vi "MultirunBuilder.vi"() -> ()   [LabVIEW 2022 SP3]
uses:
  Anemometry Sub Vis/File/Setup_Filetype.ctl
  Anemometry Sub Vis/Globals/Meas_global.vi
  Anemometry Sub Vis/Controls/Multi_run_mode.ctl
  Anemometry Sub Vis/Gen Trav/Spacing.ctl
  MultirunBuilderSubVIs/Single Measurement.vi
  MultirunBuilderSubVIs/Set Speed Only.vi
  MultirunBuilderSubVIs/Auto Calibrate.vi
  MultirunBuilderSubVIs/MoveTTcall.vi
  Anemometry Sub Vis/Controls/Tunnel_Coordinates.ctl
  MultirunBuilderSubVIs/Wait (minutes).vi
  <vilib>/Platform/system.llb/System Exec.vi
  <vilib>/Platform/browser.llb/Open URL in Default Browser (path).vi
  MultirunBuilderSubVIs/RowTemplate.ctl
  MultirunBuilderSubVIs/ReformattedTaskArray.ctl
panel:
  in  "Open Cmd File":bool
  in  "Generate Cmd File":bool
  in  "Tab Control":enum32{"Globals", "Task Array", "Dev"}(tab)
  in  "TaskArray":T1 {"Carrier_2 Q (l/min)" format="%#.2f"; "Row Duration (mins)" format="%#.1f min"; "Row No" min=0 format="row %.0f"; "Trace Gas Concentration (%)" min=0.0 format="%#_4f"; "Carrier_1 Q (l/min)" format="%#.2f"; "Tunnel Speed" format="%#.2f m/s"; "Start X" format="%#.2f"; "Start Y" format="%#.2f"; "Start Z" format="%#.2f"; "End X" format="%#.2f"; "End Y" format="%#.2f"; "End Z" format="%#.2f"; "No. of pts." format="%.0f pts"; "Averaging time (min)" min=0.0 format="%#.2f min"}
  out "Startup Index":bool
  in  "Re-initialize":bool
  in  "Stop Button":bool
  in  "RowTemplate":T3 {"Carrier_2 Q (l/min)" format="%#.2f"; "Row Duration (mins)" format="%#.1f"; "Row No" min=0; "Trace Gas Concentration (%)" min=0.0 format="%#_4f"; "Carrier_1 Q (l/min)" format="%#.2f"; "Tunnel Speed" format="%#.2f"; "Start X" format="%#.2f"; "Start Y" format="%#.2f"; "Start Z" format="%#.2f"; "End X" format="%#.2f"; "End Y" format="%#.2f"; "End Z" format="%#.2f"; "Averaging time (min)" min=0.0 format="%#.2f"}
  # "X           Y            Z"
  # "Start"
  # "End"
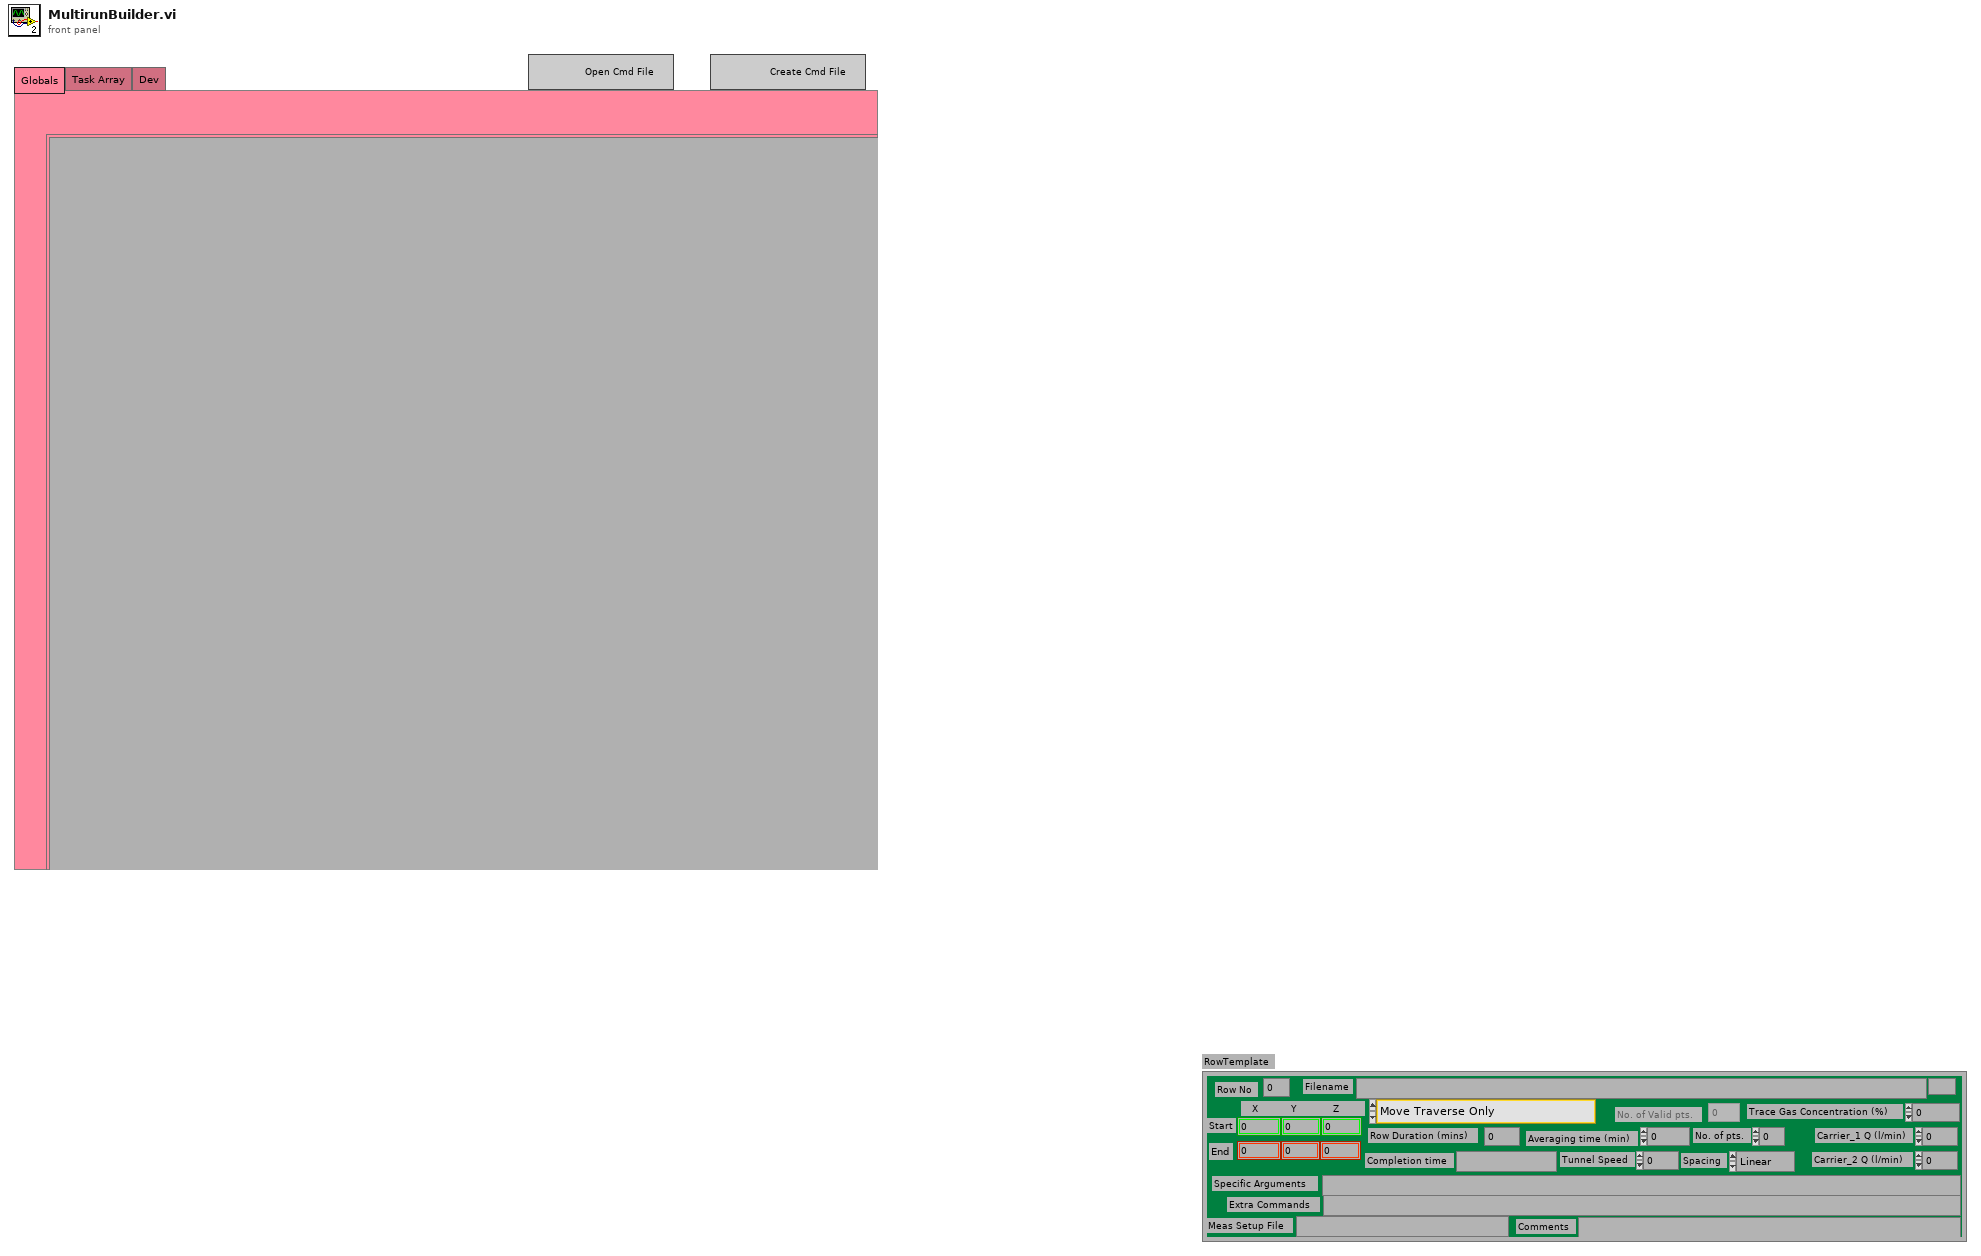
[diagram p1: front panel]
types:
  T1 = typedef "ReformattedTaskArray.ctl" = cluster{"Start X":sgl, "Start Y":sgl, "Start Z":sgl, "End X":sgl, "End Y":sgl, "End Z":sgl, "No. of pts.":i32, "Spacing":T2, "Filename":path, "Tunnel Speed":dbl, "Averaging time (min)":dbl, "Extra Commands":string, "Carrier_1 Q (l/min)":dbl, "Carrier_2 Q (l/min)":dbl, "Trace Gas Concentration (%)":dbl, "Specific Arguments":string, "Comments":string, "Row No":i32, "Row Type Selector":enum16{"Move Traverse Only", "Set Tunnel Speed Only", "Set Source Only", "Set Measurement Conditions", "Single Measurement", "Vertical Profile", "Lateral Profile", "Longitudinal Profile", "Explore Volume", "Multi-Axis Profile", "Auto Calibrate", "Meas Fast FID Bkgnd", "Check Beam Power", "Scanning Valve Measurement", "Run VI Named:", "Set ADAM Ch", "Wait (minutes)", "Send Message", "Synchronize With:", "Fall Back to this Row", "Turn Off Row Repeating", "Blank Row", "Traverse 3D Volume"}, "Completion time":string, "Row Duration (mins)":dbl, "No. of Valid pts.":i32, "Meas Setup File":string}[]
  T2 = typedef "Spacing.ctl" = enum16{"Linear", "Log", "Gauss", "Specified", "N/A"}
  T3 = typedef "RowTemplate.ctl" = cluster{"Start X":sgl, "Start Y":sgl, "Start Z":sgl, "End X":sgl, "End Y":sgl, "End Z":sgl, "No. of pts.":i32, "Spacing":T2, "Filename":path, "Tunnel Speed":dbl, "Averaging time (min)":dbl, "Extra Commands":string, "Carrier_1 Q (l/min)":dbl, "Carrier_2 Q (l/min)":dbl, "Trace Gas Concentration (%)":dbl, "Specific Arguments":string, "Comments":string, "Row No":i32, "Row Type Selector":T4, "Completion time":string, "Row Duration (mins)":dbl, "No. of Valid pts.":i32, "Meas Setup File":string}
  T4 = typedef "Multi_run_mode.ctl" = enum16{"Move Traverse Only", "Set Tunnel Speed Only", "Set Source Only", "Set Measurement Conditions", "Single Measurement", "Vertical Profile", "Lateral Profile", "Longitudinal Profile", "Multi-Axis Profile", "Explore Volume", "Auto Calibrate", "Meas Fast FID Bkgnd", "Check Beam Power", "Scanning Valve Measurement", "Run VI Named:", "Set ADAM Ch", "Wait (minutes)", "Send Message", "Synchronize With:", "Fall Back to this Row", "Turn Off Row Repeating", "Traverse 3D Volume", "Blank Row", "Jump to Fall Back Row"}
  T5 = cluster{"Azimuth Array Index":u32, "Vert Prof Array Index":u32, "Lat Prof Array Index":u32, "Azimuth Array Index 2":u32}
  T6 = enum16{"Load Command File", "Save Command File", "Check Multi Run Prog", "Check Multi Run Prog With Live Moves", "Run Multi Run Prog"}
  T7 = typedef "Tunnel_Coordinates.ctl" = enum16{"Work in Tunnel Coordinates", "Work in Model Coordinates"}
  T8 = cluster{"Tunnel Warm Up":bool, "AutoCal":bool, "Zeroes 2":bool, "Turn Table Schedule":bool, "Global Cal Checks":bool, "Local Cal Checks":bool, "Vertical Profile":bool, "Lateral Profile":bool, "Reinitialize Task Array":bool, "Save Command File":bool, "Longitudinal Profile":bool}
  T9 = typedef "CorrectionsCluster.ctl" = cluster{"Use Height Corrections":bool, "TT.Azimuths":dbl[], "Z.HeightCorrs":dbl[][], "Corrections from File":bool, "Height Survey Filepaths":path[]}
  T10 = cluster{"Start X":sgl, "Start Y":sgl, "Start Z":sgl, "End X":sgl, "End Y":sgl, "End Z":sgl, "No. of pts.":i32, "Spacing":T2, "Filename":path, "Tunnel Speed":dbl, "Averaging time (min)":dbl, "Extra Commands":string, "Carrier_1 Q (l/min)":dbl, "Carrier_2 Q (l/min)":dbl, "Trace Gas Concentration (%)":dbl, "Specific Arguments":string, "Comments":string, "Row No":i32, "Row Type Selector":T4, "Completion time":string, "Row Duration (mins)":dbl, "No. of Valid pts.":i32, "Meas Setup File":string}[]
  T11 = cluster{"Start X":sgl, "Start Y":sgl, "Start Z":sgl, "End X":sgl, "End Y":sgl, "End Z":sgl, "No. of pts.":i32, "Spacing":T2, "Filename":path, "Tunnel Speed":dbl, "Averaging time (min)":dbl, "Extra Commands":string, "Carrier_1 Q (l/min)":dbl, "Carrier_2 Q (l/min)":dbl, "Trace Gas Concentration (%)":dbl, "Specific Arguments":string, "Comments":string, "Row No":i32, "Row Type Selector":u16, "Completion time":string, "Row Duration (mins)":dbl, "No. of Valid pts.":i32, "Meas Setup File":string}[]
  T12 = typedef "SingleMeas_Repeater.ctl" = cluster{"X":dbl, "Y":dbl, "Z":dbl, "Use Tunnel Coords?":bool, "RepeatEveryXDeg":dbl}
  T13 = cluster{"Tunnel Speed":dbl, "X":dbl, "Y":dbl, "Z":dbl, "Comments":string, "Use Tunnel Coords?":bool}
  T14 = cluster{"Velocity (m/s)":dbl, "X":dbl, "Y":dbl, "Z":dbl, "Comments":string, "Use Tunnel Coords?":bool}
  T15 = typedef "MRBRowTaskSelector.ctl" = enum16{"Move Traverse Only", "Set Tunnel Speed Only", "Set Source Only", "Set Measurement Conditions", "Single Measurement", "Vertical Profile", "Lateral Profile", "Longitudinal Profile", "Explore Volume", "Multi-Axis Profile", "Auto Calibrate", "Meas Fast FID Bkgnd", "Check Beam Power", "Scanning Valve Measurement", "Run VI Named:", "MoveTT", "TravZSurvey", "Set ADAM Ch", "Wait (minutes)", "Send Message", "Synchronize With:", "Fall Back to this Row", "Turn Off Row Repeating", "Blank Row", "Traverse 3D Volume"}
  T16 = cluster{"Row Type Selector":T15, "Index":dbl, "Direction":enum16{"Forward", "Reverse"}}[]
  T17 = cluster{"Tunnel Off":bool, "Local Cal Checks":bool, "Global Cal Checks":bool, "Zeroes":bool, "AutoCal":bool, "Turn Table --> Zero":bool}
  T18 = typedef "Setup_Filetype.ctl" = enum16{"Measurement Setups", "Calibration Setups", "General", "Results File Plotter Setups", "Speed Calib Tweaks"}
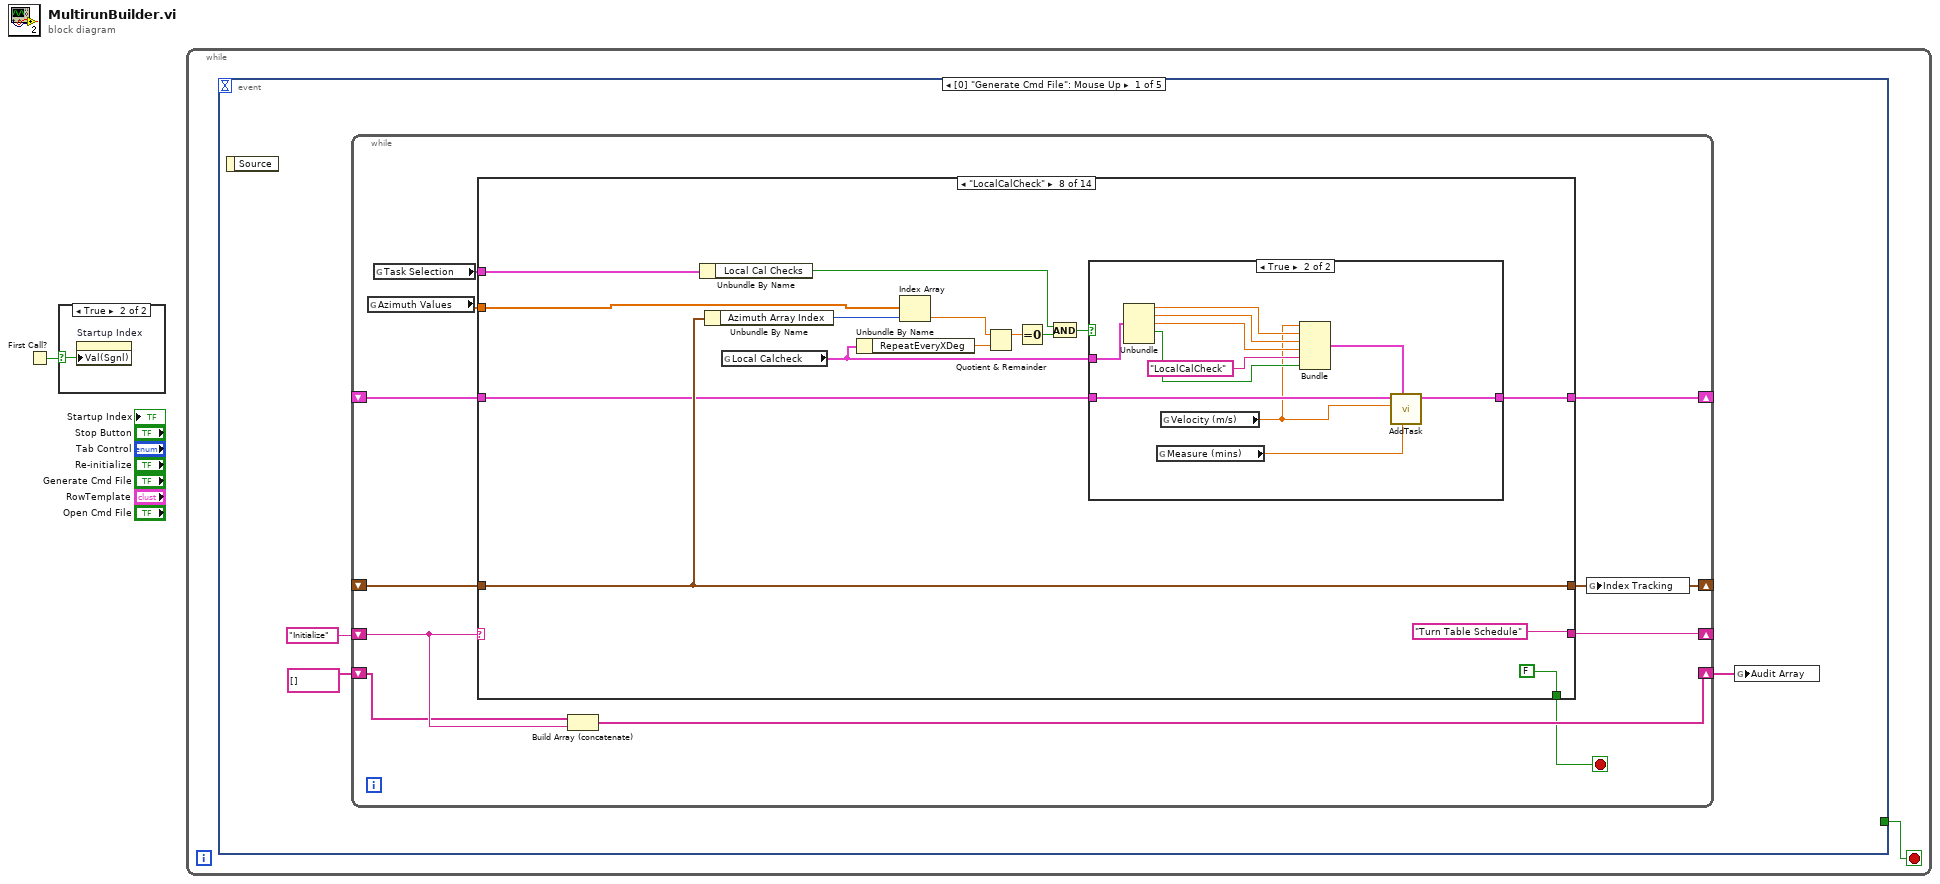
[diagram p0: block diagram]
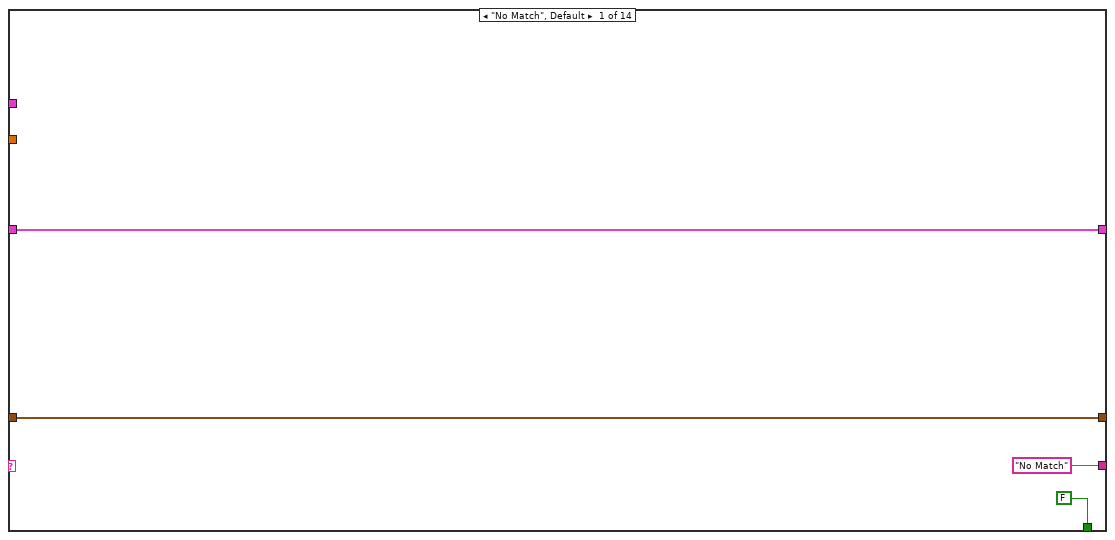
[diagram p2: hidden frame]
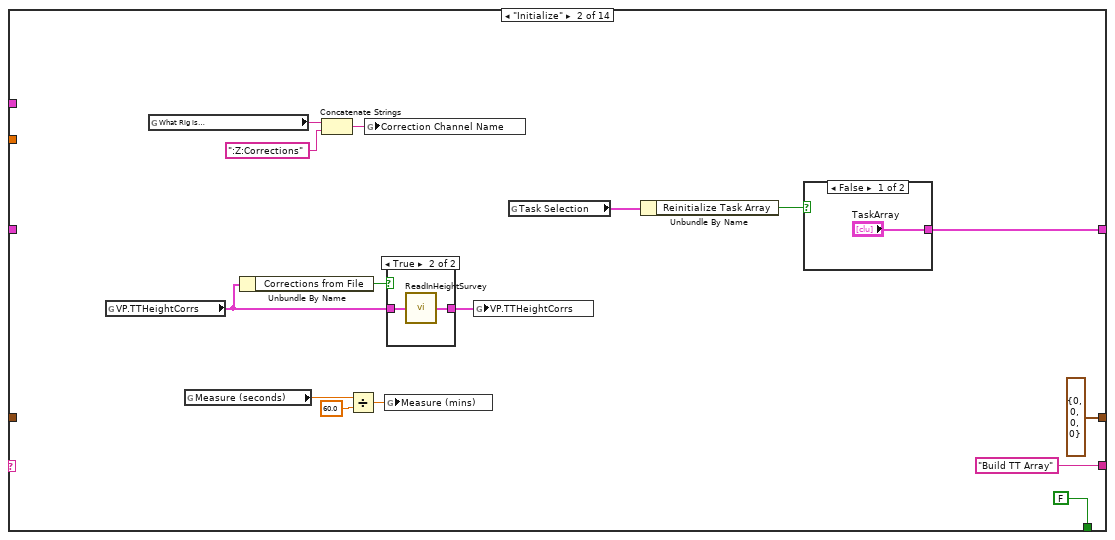
[diagram p3: hidden frame]
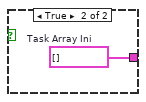
[diagram p5: hidden frame]
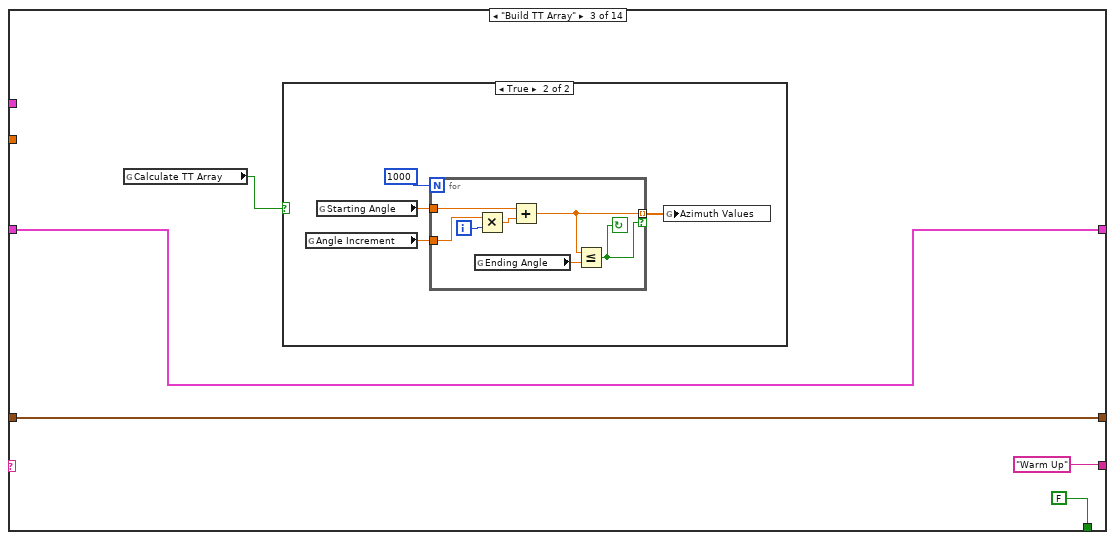
[diagram p6: hidden frame]
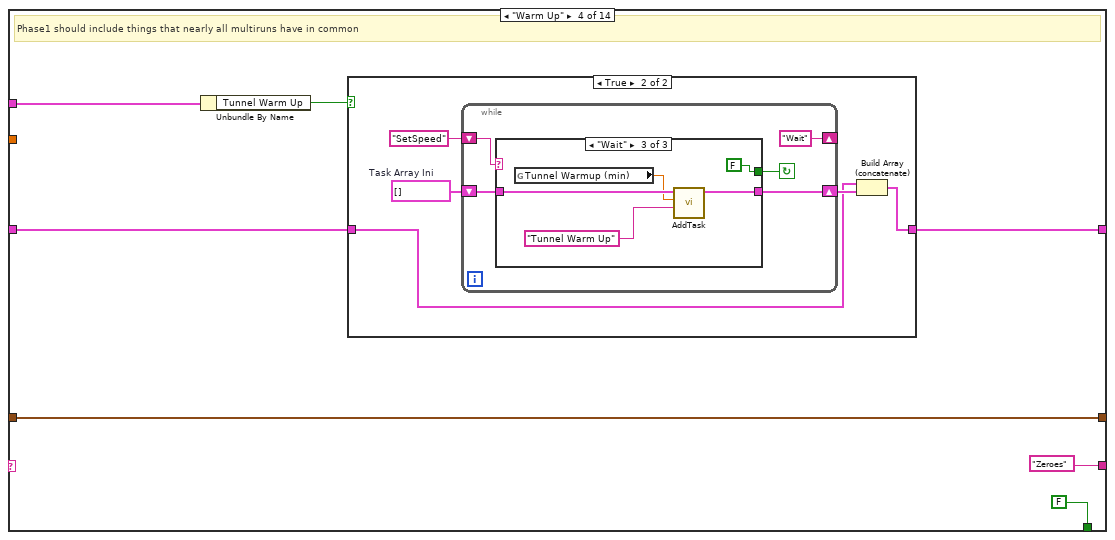
[diagram p8: hidden frame]
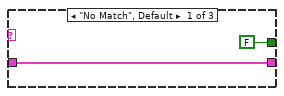
[diagram p10: hidden frame]
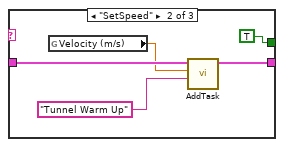
[diagram p11: hidden frame]
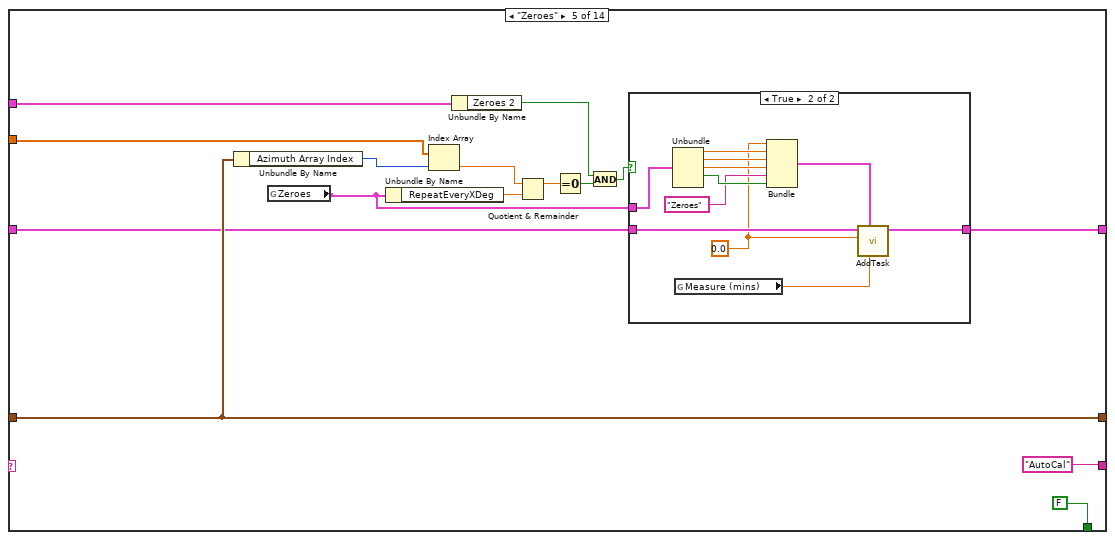
[diagram p12: hidden frame]
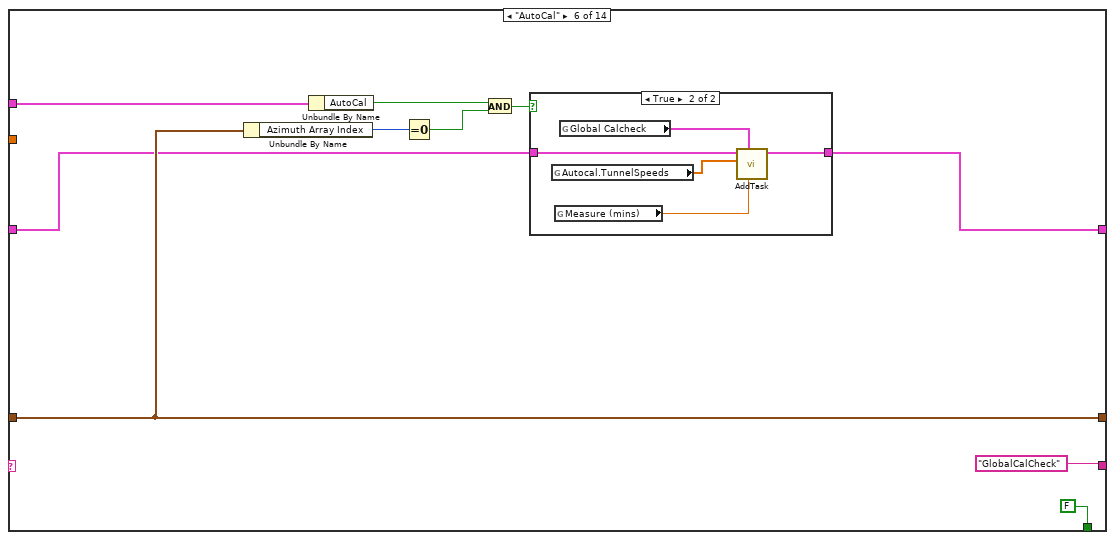
[diagram p14: hidden frame]
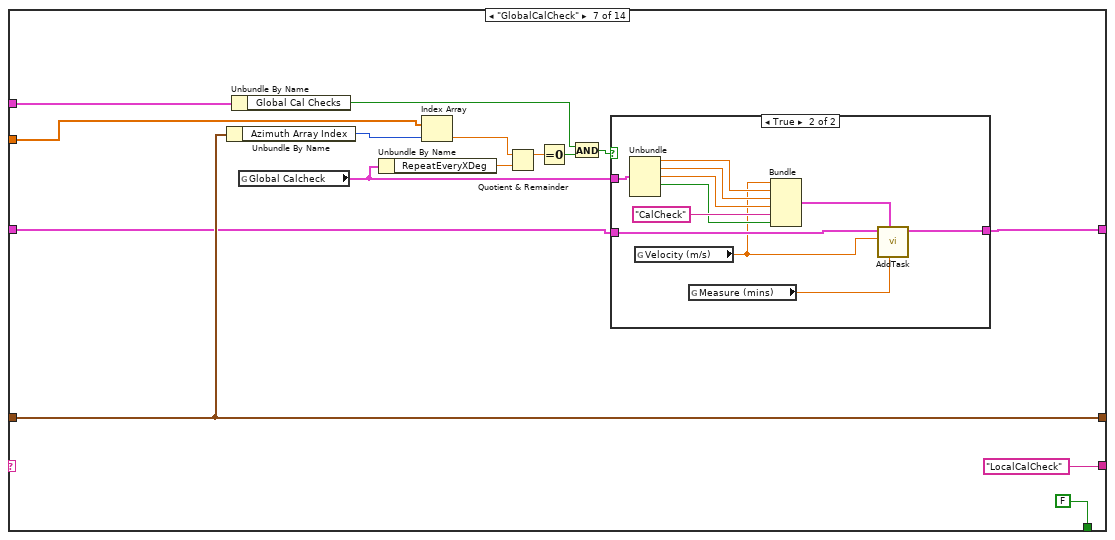
[diagram p16: hidden frame]
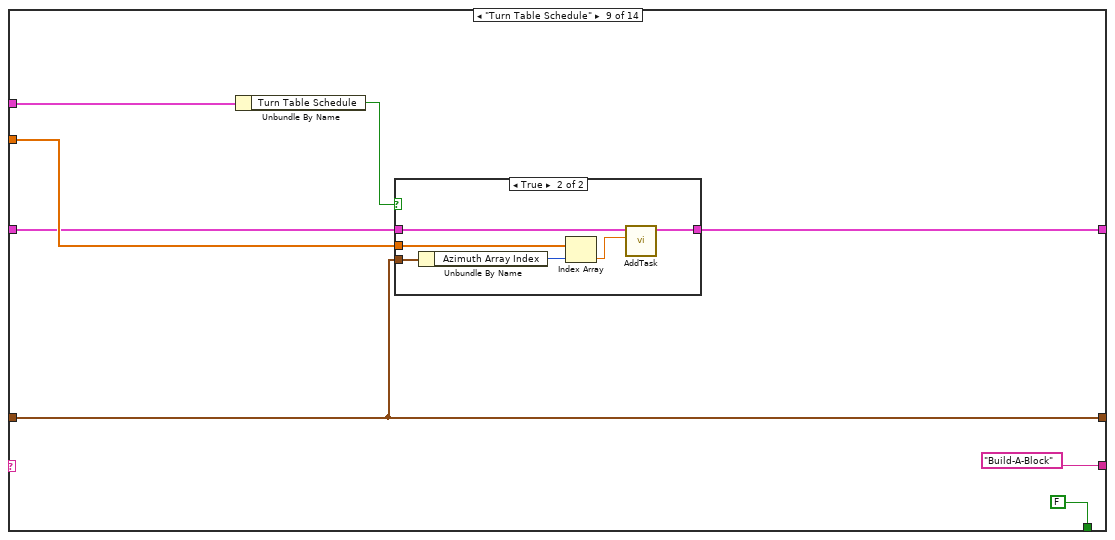
[diagram p19: hidden frame]
diagram:
  n1 = First Call?() -> (First Call?: T/F=w1:bool)
  n2 = case shown="True" w1 {
    selector: w1 -> [_ w2]
    frame False {
    }
    frame True {
      n3 = property on="Startup Index" class="Bool (strict)"("Val(Sgnl)"=w2) -> ()  [unwired: 2 in, 2 out]
    }
  }
  n4 = while {
    stop <- w3 stop-if-true
    n5 = event shown="[0] \"Generate Cmd File\": Mouse Up" {
      selector: _ -> [_ _ _ _ _]
      dyn-events: _ -> [_ _ _ _ _]
      timeout: _ -> [_ _ _ _ _]
      tunnel: [_ _ _ _ TRUE] -> w3
      event "Generate Cmd File": Mouse Up {
        n6 = event-data() -> ()  [unwired: 1 in, 1 out]
        n7 = while {
          shift-right: [w17] -> _
          shift-left: "Initialize" -> [w15]
          shift-right: [w10] -> _
          shift-left: _ -> [w11]
          shift-right: [w14] -> w6
          shift-left: string[] [] -> [w13]
          shift-right: [w9] -> _
          shift-left: _ -> [w16]
          stop <- w12 stop-if-true
          n8 = global read "MRCMDFBGlobal.vi" "Azimuth Values"() -> (w7:dbl[])
          n9 = global read "MRCMDFBGlobal.vi" "Task Selection"() -> (w8:T8)
          n10 = case shown="\"LocalCalCheck\"" w15 {
            tunnel: ["No Match" "Build TT Array" "Warm Up" "Zeroes" "AutoCal" "GlobalCalCheck" "LocalCalCheck" "Turn Table Schedule" "Build-A-Block" "Repeat?" w211 "Save Multirun?" ("t") "Last Chance for Stuff" ("t") _] -> w17
            tunnel: [FALSE ("Stop Button") FALSE ("Stop Button") FALSE ("Stop Button") FALSE ("Stop Button") FALSE ("Stop Button") FALSE ("Stop Button") FALSE ("Stop Button") FALSE ("Stop Button") FALSE ("Stop Button") FALSE ("Stop Button") FALSE ("Stop Button") FALSE FALSE TRUE ("Stop Button")] -> w12
            tunnel: w7 -> [_ _ _ _ w100 _ w135 w161 w191 _ w210 _ _ _]
            tunnel: w16 -> [w19 _ w45 w62 w98 w121 w138 w166 w187 w201 w216 w244 w342 w364]
            tunnel: [w19 T5 {"Azimuth Array Index"=0, "Vert Prof Array Index"=0, "Lat Prof Array Index"=0, "Azimuth Array Index 2"=0} ("Index Tracking") w45 w62 w98 w121 w138 w166 w187 w201 w214 w244 w342 w364] -> w9
            tunnel: w8 -> [_ _ _ w61 w94 w117 w137 w165 w188 _ w207 _ w346 _]
            tunnel: w11 -> [w18 _ w43 w59 w89 w115 w132 w160 w186 w203 w208 w235 w344 w363]
            tunnel: [w18 w31 w43 w58 w90 w116 w133 w159 w185 w202 w208 w236 w340 w363] -> w10
            frame "No Match", Default {
            }
            frame "Initialize" {
              n11 = global read "MRCMDFBGlobal.vi" "VP.TTHeightCorrs"() -> (w28:T9)
              n12 = global read "MRCMDFBGlobal.vi" "What Rig is\nMultirunning?"() -> (w24:string)
              n13 = global read "MRCMDFBGlobal.vi" "Measure (seconds)"() -> (w25:dbl)
              n14 = Unbundle By Name(w28) -> ("Corrections from File"=w30:bool)
              n15 = Concatenate Strings(w24, ":Z:Corrections") -> (w22:string)
              n16 = Divide(x=w25, y=60.0 ("x")) -> (x/y=w26:dbl)
              n17 = global write "MRCMDFBGlobal.vi" "Correction Channel Name"(w22) -> ()
              n18 = global write "MRCMDFBGlobal.vi" "Measure (mins)"(w26) -> ()
              n19 = case shown="True" w30 {
                tunnel: w28 -> [w37 w39]
                tunnel: [w37 w38] -> w29
                frame False {
                }
                frame True {
                  n20 = call "ReadInHeightSurvey.vi"("VP.TTHeightCorrs In"=w39) -> ("VP.TTHeightCorrs Out"=w38:T9)
                }
              }
              n21 = global write "MRCMDFBGlobal.vi" "VP.TTHeightCorrs"(w29) -> ()
              n22 = global read "MRCMDFBGlobal.vi" "Task Selection"() -> (w33:T8)
              n23 = Unbundle By Name(w33) -> ("Reinitialize Task Array"=w32:bool)
              n24 = case shown="False" w32 {
                tunnel: ["TaskArray" w41] -> w31
                frame False {
                }
                frame True {
                  w41 = T10 []  # Task Array Ini
                }
              }
            }
            frame "Build TT Array" {
              n25 = global read "MRCMDFBGlobal.vi" "Calculate TT Array"() -> (w42:bool)
              n26 = case shown="True" w42 {
                frame False {
                }
                frame True {
                  n27 = global read "MRCMDFBGlobal.vi" "Angle Increment"() -> (w47:dbl)
                  n28 = global read "MRCMDFBGlobal.vi" "Starting Angle"() -> (w48:dbl)
                  n29 = for {
                    N: 1000 -> [_]
                    tunnel: w48 -> [w55]
                    tunnel: w47 -> [w56]
                    tunnel: [w53] -> w49 mode=indexing if=w52
                    i -> [w57]
                    stop <- w52 continue-if-true
                    n30 = global read "MRCMDFBGlobal.vi" "Ending Angle"() -> (w51:dbl)
                    n31 = Multiply(x=w56, y=w57) -> (x*y=w54:dbl)
                    n32 = Add(x=w55, y=w54) -> (x+y=w53:dbl)
                    n33 = Less Or Equal?(x=w53, y=w51) -> (x <= y?=w52:bool)
                  }
                  n34 = global write "MRCMDFBGlobal.vi" "Azimuth Values"(w49) -> ()
                }
              }
            }
            frame "Warm Up" {
              # "Phase1 should include things that nearly all multiruns have in common"
              n35 = Unbundle By Name(w61) -> ("Tunnel Warm Up"=w60:bool)
              n36 = case shown="True" w60 {
                tunnel: w59 -> [w65 w67]
                tunnel: [w65 w66] -> w58
                frame False {
                }
                frame True {
                  w69 = T10 []  # Task Array Ini
                  n37 = while {
                    shift-right: ["Wait"] -> _
                    shift-left: "SetSpeed" -> [w75]
                    shift-right: [w71] -> w68
                    shift-left: w69 -> [w72]
                    stop <- w73 continue-if-true
                    n38 = case shown="\"Wait\"" w75 {
                      tunnel: [FALSE TRUE FALSE] -> w73
                      tunnel: w72 -> [w76 w80 w85]
                      tunnel: [w76 w79 w84] -> w71
                      frame "No Match", Default {
                      }
                      frame "SetSpeed" {
                        n39 = global read "MRCMDFBGlobal.vi" "Velocity (m/s)"() -> (w78:dbl)
                        n40 = call-poly "AddTask.vi"("Comments"="Tunnel Warm Up", "Tunnel Speed"=w78, "Input Task Array"=w80) -> ("Output Task Array"=w79:T3[])  [unwired: 8 in]
                      }
                      frame "Wait" {
                        n41 = global read "MRCMDFBGlobal.vi" "Tunnel Warmup (min)"() -> (w83:dbl)
                        n42 = call-poly "AddTask.vi"("Comments"="Tunnel Warm Up", "Wait Time (min)"=w83, "Input Task Array"=w85) -> ("Output Task Array"=w84:T3[])  [unwired: 8 in]
                      }
                    }
                  }
                  n43 = Build Array (concatenate)(w67, w68) -> (w66:T11)
                }
              }
            }
            frame "Zeroes" {
              n44 = Unbundle By Name(w98) -> ("Azimuth Array Index"=w99:u32)
              n45 = global read "MRCMDFBGlobal.vi" "Zeroes"() -> (w88:T12)
              n46 = Unbundle By Name(w88) -> ("RepeatEveryXDeg"=w96:dbl)
              n47 = Index Array(array=w100, index=w99) -> (element=w97:dbl)
              n48 = Unbundle By Name(w94) -> ("Zeroes 2"=w93:bool)
              n49 = Quotient & Remainder(x=w97, y=w96) -> (x-y*floor(x/y)=w95:dbl)  [unwired: 1 out]
              n50 = Equal To 0?(x=w95) -> (x = 0?=w92:bool)
              n51 = And(x=w93, y=w92) -> (x .and. y?=w91:bool)
              n52 = case shown="True" w91 {
                tunnel: w88 -> [_ w112]
                tunnel: [w103 w114] -> w90
                tunnel: w89 -> [w103 w113]
                frame False {
                }
                frame True {
                  w104 = 0.0 ("Tunnel Speed")
                  n53 = Unbundle(w112) -> ("X"=w111:dbl, "Y"=w110:dbl, "Z"=w109:dbl, "Use Tunnel Coords?"=w107:bool)  [unwired: 1 out]
                  n54 = global read "MRCMDFBGlobal.vi" "Measure (mins)"() -> (w105:dbl)
                  n55 = Bundle("Tunnel Speed"=w104, "X"=w111, "Y"=w110, "Z"=w109, "Comments"="Zeroes", "Use Tunnel Coords?"=w107) -> (w108:T13)  [unwired: 1 in]
                  n56 = call-poly "AddTask.vi"("Averaging time (min)"=w105, "Coordinate Description"=w108, "Tunnel Speed"=w104, "Input Task Array"=w113) -> ("Output Task Array"=w114:T3[])  [unwired: 7 in]
                }
              }
            }
            frame "AutoCal" {
              n57 = Unbundle By Name(w121) -> ("Azimuth Array Index"=w120:u32)
              n58 = Unbundle By Name(w117) -> ("AutoCal"=w119:bool)
              n59 = Equal To 0?(x=w120) -> (x = 0?=w122:bool)
              n60 = And(x=w119, y=w122) -> (x .and. y?=w118:bool)
              n61 = case shown="True" w118 {
                tunnel: [w125 w130] -> w116
                tunnel: w115 -> [w125 w129]
                frame False {
                }
                frame True {
                  n62 = global read "MRCMDFBGlobal.vi" "Autocal.TunnelSpeeds"() -> (w128:dbl[])
                  n63 = global read "MRCMDFBGlobal.vi" "Measure (mins)"() -> (w127:dbl)
                  n64 = global read "MRCMDFBGlobal.vi" "Global Calcheck"() -> (w126:T12)
                  n65 = call-poly "AddTask.vi"("Averaging time (min)"=w127, "Global Calcheck"=w126, "Autocal.TunnelSpeeds"=w128, "Input Task Array"=w129) -> ("Output Task Array"=w130:T3[])  [unwired: 7 in]
                }
              }
            }
            frame "GlobalCalCheck" {
              n66 = Unbundle By Name(w138) -> ("Azimuth Array Index"=w143:u32)
              n67 = Unbundle By Name(w137) -> ("Global Cal Checks"=w136:bool)
              n68 = global read "MRCMDFBGlobal.vi" "Global Calcheck"() -> (w131:T12)
              n69 = Unbundle By Name(w131) -> ("RepeatEveryXDeg"=w141:dbl)
              n70 = Index Array(array=w135, index=w143) -> (element=w142:dbl)
              n71 = Quotient & Remainder(x=w142, y=w141) -> (x-y*floor(x/y)=w140:dbl)  [unwired: 1 out]
              n72 = Equal To 0?(x=w140) -> (x = 0?=w139:bool)
              n73 = And(x=w136, y=w139) -> (x .and. y?=w134:bool)
              n74 = case shown="True" w134 {
                tunnel: w131 -> [_ w155]
                tunnel: [w146 w157] -> w133
                tunnel: w132 -> [w146 w156]
                frame False {
                }
                frame True {
                  n75 = Unbundle(w155) -> ("X"=w153:dbl, "Y"=w152:dbl, "Z"=w151:dbl, "Use Tunnel Coords?"=w150:bool)  [unwired: 1 out]
                  n76 = global read "MRCMDFBGlobal.vi" "Velocity (m/s)"() -> (w147:dbl)
                  n77 = global read "MRCMDFBGlobal.vi" "Measure (mins)"() -> (w148:dbl)
                  n78 = Bundle("Velocity (m/s)"=w147, "X"=w153, "Y"=w152, "Z"=w151, "Comments"="CalCheck", "Use Tunnel Coords?"=w150) -> (w149:T14)  [unwired: 1 in]
                  n79 = call-poly "AddTask.vi"("Averaging time (min)"=w148, "Coordinate Description"=w149, "Tunnel Speed"=w147, "Input Task Array"=w156) -> ("Output Task Array"=w157:T3[])  [unwired: 7 in]
                }
              }
            }
            frame "LocalCalCheck" {
              n80 = Unbundle By Name(w165) -> ("Local Cal Checks"=w164:bool)
              n81 = Unbundle By Name(w166) -> ("Azimuth Array Index"=w170:u32)
              n82 = global read "MRCMDFBGlobal.vi" "Local Calcheck"() -> (w158:T12)
              n83 = Unbundle By Name(w158) -> ("RepeatEveryXDeg"=w168:dbl)
              n84 = Index Array(array=w161, index=w170) -> (element=w169:dbl)
              n85 = Quotient & Remainder(x=w169, y=w168) -> (x-y*floor(x/y)=w167:dbl)  [unwired: 1 out]
              n86 = Equal To 0?(x=w167) -> (x = 0?=w163:bool)
              n87 = And(x=w164, y=w163) -> (x .and. y?=w162:bool)
              n88 = case shown="True" w162 {
                tunnel: w158 -> [_ w182]
                tunnel: w160 -> [w173 w184]
                tunnel: [w173 w183] -> w159
                frame False {
                }
                frame True {
                  n89 = Unbundle(w182) -> ("X"=w176:dbl, "Y"=w177:dbl, "Z"=w178:dbl, "Use Tunnel Coords?"=w179:bool)  [unwired: 1 out]
                  n90 = global read "MRCMDFBGlobal.vi" "Measure (mins)"() -> (w175:dbl)
                  n91 = global read "MRCMDFBGlobal.vi" "Velocity (m/s)"() -> (w174:dbl)
                  n92 = Bundle("Velocity (m/s)"=w174, "X"=w176, "Y"=w177, "Z"=w178, "Comments"="LocalCalCheck", "Use Tunnel Coords?"=w179) -> (w180:T14)  [unwired: 1 in]
                  n93 = call-poly "AddTask.vi"("Averaging time (min)"=w175, "Coordinate Description"=w180, "Tunnel Speed"=w174, "Input Task Array"=w184) -> ("Output Task Array"=w183:T3[])  [unwired: 7 in]
                }
              }
            }
            frame "Turn Table Schedule" {
              n94 = Unbundle By Name(w188) -> ("Turn Table Schedule"=w189:bool)
              n95 = case shown="True" w189 {
                tunnel: w191 -> [_ w199]
                tunnel: w187 -> [_ w198]
                tunnel: w186 -> [w193 w197]
                tunnel: [w193 w196] -> w185
                frame False {
                }
                frame True {
                  n96 = Unbundle By Name(w198) -> ("Azimuth Array Index"=w195:u32)
                  n97 = Index Array(array=w199, index=w195) -> (element=w194:dbl)
                  n98 = call-poly "AddTask.vi"("TT:Azimuth"=w194, "Input Task Array"=w197) -> ("Output Task Array"=w196:T3[])  [unwired: 9 in]
                }
              }
            }
            frame "Build-A-Block" {
              n99 = global read "MRCMDFBGlobal.vi" "Build-A-Block"() -> (w200:T16)
              n100 = call "MR_Build-A-Block.vi"("Build-A-Block"=w200) -> ("TaskArray"=w204:T10)
              n101 = Build Array (concatenate)(w203, w204) -> (w202:T11)
            }
            frame "Repeat?" {
              # "Only reason to repeat is if TT Scheduling"
              n102 = Unbundle By Name(w207) -> ("Turn Table Schedule"=w209:bool)
              n103 = case shown="True" w209 {
                tunnel: w216 -> [w218 w225]
                tunnel: [TRUE w224] -> w215
                tunnel: [w218 w223] -> w214
                tunnel: w210 -> [_ w222]
                frame False {
                }
                frame True {
                  n104 = Array Size(array=w222) -> (size(s)=w221:i32)
                  n105 = Decrement(x=w221) -> (x-1=w220:i32)
                  n106 = in-place {
                    in-place-border: w220 -> [w227]
                    in-place-border: [w228] -> w224
                    n107 = in-place-cluster #1(w225) -> ("Azimuth Array Index"=w226:u32)
                    n108 = Equal?(x=w227, y=w226) -> (x = y?=w228:bool)
                    n109 = case shown="True" w228 {
                      tunnel: [w230 0] -> w229
                      tunnel: w226 -> [w231 _]
                      frame False {
                        n110 = Increment(x=w231) -> (x+1=w230:u32)
                      }
                      frame True {
                      }
                    }
                    n111 = in-place-cluster #1("Azimuth Array Index"=w229) -> (w223:T5)
                  }
                }
              }
              n112 = Select(t="End", s=w215, f="Zeroes" ("t")) -> (s? t:f=w211:string)
            }
            frame "End" {
              n113 = global read "MRCMDFBGlobal.vi" "Multirun Closure Tasks"() -> (w233:T17)
              n114 = Unbundle By Name(w233) -> ("Turn Table --> Zero"=w242:bool, "Zeroes"=w241:bool, "AutoCal"=w240:bool, "Global Cal Checks"=w239:bool, "Local Cal Checks"=w238:bool, "Tunnel Off"=w237:bool)
              n115 = while {
                shift-right: [w255] -> _
                shift-left: "Turn Table" -> [w256]
                tunnel: w242 -> [w254]
                tunnel: w241 -> [w251]
                tunnel: w240 -> [w250]
                tunnel: w239 -> [w249]
                tunnel: w238 -> [w248]
                tunnel: w237 -> [w247]
                shift-right: [w252] -> w236
                shift-left: w235 -> [w253]
                stop <- w246 continue-if-true
                n116 = case shown="\"Zeroes\"" w256 {
                  tunnel: [_ "Zeroes" "AutoCal" "GlobalCalCheck" "LocalCalCheck" "Tunnel Off" _] -> w255
                  tunnel: w254 -> [_ w263 _ _ _ _ _]
                  tunnel: w253 -> [w258 w262 w272 w289 w300 w317 w333]
                  tunnel: [w258 w261 w271 w288 w299 w316 w332] -> w252
                  tunnel: w251 -> [_ _ w268 _ _ _ _]
                  tunnel: w250 -> [_ _ _ w285 _ _ _]
                  tunnel: w249 -> [_ _ _ _ w297 _ _]
                  tunnel: w248 -> [_ _ _ _ _ w314 _]
                  tunnel: w247 -> [_ _ _ _ _ _ w331]
                  tunnel: [FALSE TRUE TRUE TRUE TRUE TRUE TRUE] -> w246
                  frame "No Match", Default {
                  }
                  frame "Turn Table" {
                    n117 = case shown="True" w263 {
                      tunnel: w262 -> [w264 w266]
                      tunnel: [w264 w265] -> w261
                      frame False {
                      }
                      frame True {
                        n118 = call-poly "AddTask.vi"("TT:Azimuth"=0.0, "Input Task Array"=w266) -> ("Output Task Array"=w265:T3[])  [unwired: 9 in]
                      }
                    }
                  }
                  frame "Zeroes" {
                    n119 = case shown="True" w268 {
                      tunnel: w272 -> [w273 w284]
                      tunnel: [w273 w283] -> w271
                      frame False {
                      }
                      frame True {
                        w274 = 0.0 ("Tunnel Speed")
                        n120 = global read "MRCMDFBGlobal.vi" "Zeroes"() -> (w275:T12)
                        n121 = global read "MRCMDFBGlobal.vi" "Measure (mins)"() -> (w276:dbl)
                        n122 = Unbundle(w275) -> ("X"=w281:dbl, "Y"=w280:dbl, "Z"=w279:dbl, "Use Tunnel Coords?"=w278:bool)  [unwired: 1 out]
                        n123 = Bundle("Tunnel Speed"=w274, "X"=w281, "Y"=w280, "Z"=w279, "Comments"="Zeroes", "Use Tunnel Coords?"=w278) -> (w277:T13)  [unwired: 1 in]
                        n124 = call-poly "AddTask.vi"("Averaging time (min)"=w276, "Coordinate Description"=w277, "Tunnel Speed"=w274, "Input Task Array"=w284) -> ("Output Task Array"=w283:T3[])  [unwired: 7 in]
                      }
                    }
                  }
                  frame "AutoCal" {
                    n125 = case shown="True" w285 {
                      tunnel: w289 -> [w290 w295]
                      tunnel: [w290 w294] -> w288
                      frame False {
                      }
                      frame True {
                        n126 = global read "MRCMDFBGlobal.vi" "Autocal.TunnelSpeeds"() -> (w293:dbl[])
                        n127 = global read "MRCMDFBGlobal.vi" "Global Calcheck"() -> (w291:T12)
                        n128 = global read "MRCMDFBGlobal.vi" "Measure (mins)"() -> (w292:dbl)
                        n129 = call-poly "AddTask.vi"("Averaging time (min)"=w292, "Global Calcheck"=w291, "Autocal.TunnelSpeeds"=w293, "Input Task Array"=w295) -> ("Output Task Array"=w294:T3[])  [unwired: 7 in]
                      }
                    }
                  }
                  frame "GlobalCalCheck" {
                    n130 = case shown="True" w297 {
                      tunnel: w300 -> [w301 w312]
                      tunnel: [w301 w311] -> w299
                      frame False {
                      }
                      frame True {
                        n131 = global read "MRCMDFBGlobal.vi" "Global Calcheck"() -> (w304:T12)
                        n132 = global read "MRCMDFBGlobal.vi" "Measure (mins)"() -> (w303:dbl)
                        n133 = global read "MRCMDFBGlobal.vi" "Velocity (m/s)"() -> (w302:dbl)
                        n134 = Unbundle(w304) -> ("X"=w308:dbl, "Y"=w307:dbl, "Z"=w306:dbl, "Use Tunnel Coords?"=w305:bool)  [unwired: 1 out]
                        n135 = Bundle("Velocity (m/s)"=w302, "X"=w308, "Y"=w307, "Z"=w306, "Comments"="CalCheck", "Use Tunnel Coords?"=w305) -> (w309:T14)  [unwired: 1 in]
                        n136 = call-poly "AddTask.vi"("Averaging time (min)"=w303, "Coordinate Description"=w309, "Tunnel Speed"=w302, "Input Task Array"=w312) -> ("Output Task Array"=w311:T3[])  [unwired: 7 in]
                      }
                    }
                  }
                  frame "LocalCalCheck" {
                    n137 = case shown="True" w314 {
                      tunnel: w317 -> [w318 w329]
                      tunnel: [w318 w328] -> w316
                      frame False {
                      }
                      frame True {
                        n138 = global read "MRCMDFBGlobal.vi" "Local Calcheck"() -> (w321:T12)
                        n139 = global read "MRCMDFBGlobal.vi" "Velocity (m/s)"() -> (w319:dbl)
                        n140 = global read "MRCMDFBGlobal.vi" "Measure (mins)"() -> (w320:dbl)
                        n141 = Unbundle(w321) -> ("X"=w327:dbl, "Y"=w326:dbl, "Z"=w325:dbl, "Use Tunnel Coords?"=w322:bool)  [unwired: 1 out]
                        n142 = Bundle("Velocity (m/s)"=w319, "X"=w327, "Y"=w326, "Z"=w325, "Comments"="LocalCalCheck", "Use Tunnel Coords?"=w322) -> (w323:T14)  [unwired: 1 in]
                        n143 = call-poly "AddTask.vi"("Averaging time (min)"=w320, "Coordinate Description"=w323, "Tunnel Speed"=w319, "Input Task Array"=w329) -> ("Output Task Array"=w328:T3[])  [unwired: 7 in]
                      }
                    }
                  }
                  frame "Tunnel Off" {
                    n144 = case shown="True" w331 {
                      tunnel: w333 -> [w334 w336]
                      tunnel: [w334 w335] -> w332
                      frame False {
                      }
                      frame True {
                        n145 = call-poly "AddTask.vi"("Comments"="Tunnel Off", "Tunnel Speed"=0.0, "Input Task Array"=w336) -> ("Output Task Array"=w335:T3[])  [unwired: 8 in]
                      }
                    }
                  }
                }
              }
            }
            frame "Save Multirun?" {
              n146 = Unbundle By Name(w346) -> ("Save Command File"=w345:bool)
              n147 = global read "MRCMDFBGlobal.vi" "Command File Path / Name"() -> (w341:path)
              n148 = case shown="True" w345 {
                tunnel: w341 -> [_ w352]
                tunnel: w344 -> [w347 w349]
                tunnel: [w347 w349] -> w340
                frame False {
                }
                frame True {
                  n149 = global read "MRCMDFBGlobal.vi" "Work in TUNNEL Coordinates"() -> (w348:bool)
                  n150 = case shown="False" w348 {
                    tunnel: [Tunnel_Coordinates."Work in Model Coordinates" ("Work in Tunnel Coordinates?") Tunnel_Coordinates."Work in Tunnel Coordinates" ("Work in Tunnel Coordinates?")] -> w350
                    frame False {
                    }
                    frame True {
                    }
                  }
                  n151 = call "Multi_Run_Prog.vi"("Command filename"=w352, "Mode"=T6."Save Command File", "Table"=w349, "Work in Tunnel Coordinates?"=w350) -> ()  [unwired: 15 in, 1 out]
                }
              }
              n152 = local write "TaskArray"(w340) -> ()
            }
            frame "Last Chance for Stuff" {
              n153 = vi-ref "Multi_Run_Prog.vi"() -> (w356:refnum<vi>)
              n154 = property class="VI"(reference=w356) -> (error out=w359:errorcluster, "Panel"=w357:refnum<vi>)  [unwired: 1 in, 1 out]
              n155 = property class="Pnl"(reference=w357, error in=w359) -> (error out=w360:errorcluster, "Controls[]"=w358:refnum<vi>[])  [unwired: 1 out]
              n156 = for {
                tunnel: w358 -> [w370] mode=indexing
                tunnel: [w369] -> w361 if=w368
                tunnel: w360 -> [w367]
                stop <- w368 stop-if-true
                n157 = property class="Ctl"(reference=w370, error in=w367) -> (reference out=w371:refnum<vi>, error out=w366:errorcluster, "Label.Text"=w372:string)
                n158 = property class="Ctl"(reference=w371, error in=w366) -> ("Value"=w369:variant)  [unwired: 2 out]
                n159 = Equal?(x=w372, y="Command filename") -> (x = y?=w368:bool)
              }
              n160 = Variant To Data(type=path "", Variant=w361) -> (data=w355:path)  [unwired: 1 in, 1 out]
              n161 = global write "MRCMDFBGlobal.vi" "Command File Path / Name"(w355) -> ()
            }
          }
          n162 = Build Array (concatenate)(w13, w15) -> (w14:string[])
          n163 = global write "MRCMDFBGlobal.vi" "Index Tracking"(w9) -> ()
        }
        n164 = global write "MRCMDFBGlobal.vi" "Audit Array"(w6) -> ()
      }
      event "Re-initialize": Mouse Up; "Startup Index": Value Change {
        n165 = event-data() -> ()  [unwired: 1 in, 4 out]
        n166 = while {
          shift-right: [w376] -> _
          shift-left: "Load Subpanel" -> [w377]
          stop <- w375 stop-if-true
          n167 = case shown="\"Meas Setups\"" w377 {
            tunnel: ["End" "End" "End" "Meas Setups"] -> w376
            tunnel: [TRUE _ TRUE _] -> w375
            frame "No Match", Default {
            }
            frame "Meas Setups" {
              n168 = disable-structure shown="Enabled" {
                frame Disabled {
                  w383 = Setup_Filetype."Measurement Setups" ("Setup File Type")
                  w388 = string[] [] ("file names")
                  n169 = call "Last_Years_Setups.vi"("Setup File Type"=w383) -> ("Directory"=w382:path)
                  n170 = call "Setup_Filepath.vi"("Setup File Type"=w383, "Filename in"="Test") -> ("Directory"=w384:path)  [unwired: 1 out]
                  n171 = call "List_files_in_order_of_age.vi"("Files to Hide"=w388, "Folder"=w384) -> ("file names"=w385:string[])
                  n172 = call "List_files_in_order_of_age.vi"("Files to Hide"=w388, "Folder"=w382) -> ("file names"=w386:string[])
                  n173 = Build Array (concatenate)(w385, w386) -> ()  [unwired: 1 out]
                }
                frame Enabled {
                }
              }
              n174 = global write "Meas_global.vi" "Remote control"(FALSE ("Remote control")) -> ()
            }
            frame "End" {
            }
            frame "Load Subpanel" {
              n175 = property on="MRCMDFBGlobals" class="SubPnl"() -> (error out=w391:errorcluster, "InsertedVI"=w393:refnum<vi>)  [unwired: 2 in, 1 out]
              n176 = Not A Number/Path/Refnum?(number/path/refnum=w393) -> (NaN/Path/Refnum?=w392:bool)
              n177 = case shown="True" w392 {
                tunnel: w391 -> [_ w395]
                frame False {
                }
                frame True {
                  n178 = vi-ref "MRCMDFBGlobal.vi"() -> (w396:refnum<vi>)
                  n179 = invoke on="MRCMDFBGlobals" class="SubPnl" method="Insert VI"(error in=w395, "VI Ref"=w396) -> ()  [unwired: 2 in, 4 out]
                }
              }
            }
          }
        }
      }
      event Timeout {
        n180 = event-data() -> ()  [unwired: 1 in, 3 out]
      }
      event "Open Cmd File": Mouse Up {
        n181 = event-data() -> ()  [unwired: 1 in, 1 out]
        n182 = global read "MRCMDFBGlobal.vi" "Command File Path / Name"() -> (w398:path)
        n183 = call "Does_file_exist_(simple).vi"("Pathname"=w398) -> ("exists?"=w397:bool)
        n184 = case shown="True" w397 {
          tunnel: w398 -> [w402 w403]
          frame False {
            n185 = Path To String(path=w402) -> (string=w400:string)
            n186 = Concatenate Strings("File does not exist :\n" ("string"), w400) -> (w399:string)
            n187 = One Button Dialog(message=w399) -> ()  [unwired: 1 in, 1 out]
          }
          frame True {
            n188 = disable-structure shown="Enabled" {
              disable-tunnel: w403 -> [w407 w410]
              frame Enabled {
                n189 = Strip Path(path=w407) -> (stripped path=w409:path, name=w405:string)
                n190 = Concatenate Strings("cmd /c", w405) -> (w404:string)
                n191 = call "5060002"("wait until completion? (T)"=FALSE, "working directory"=w409, "command line"=w404) -> ()  [unwired: 5 in, 4 out]
              }
              frame Disabled {
                n192 = call-poly <vilib>:"Open URL in Default Browser.vi"("path"=w410) -> ()  [unwired: 5 in, 2 out]
              }
            }
          }
        }
      }
      event "Stop Button": Mouse Up; Panel Close {
        n193 = event-data() -> ()  [unwired: 1 in, 3 out]
        n194 = invoke on="MRCMDFBGlobals" class="SubPnl" method="Remove VI"() -> ()  [unwired: 3 in, 3 out]
      }
    }
  }
